vi "Receive Signal DBL.vi"(8 "error in":errorcluster, 10 "Signal Name":string, 11 "DBC Communication in":refnum<class "DBC Communicator.lvclass">) -> (0 "error out":errorcluster, 1 "Time Stamp":timestamp format="%<%x %.3X>T", 2 "Value":dbl, 3 "DBC Communication out":refnum<class "DBC Communicator.lvclass">)   [LabVIEW 2025, in "DBC Communicator.lvclass"]
uses:
  DBC Communicator.lvclass
  <vilib>/xnet/xnet.llb/XNET Frame Type CAN.ctl
  <vilib>/Utility/miscctls.llb/LVMapReplaceAction.ctl
  c9a96274-a027-4ccf-b481-50e0b552ac68.vi
  <vilib>/Utility/error.llb/Trim Whitespace One-Sided.vi
  c9a96274-a027-4ccf-b481-50e0b552ac68.vi/d4db2432-cc9c-482c-8957-dac855435ef6.vi
  c9a96274-a027-4ccf-b481-50e0b552ac68.vi/86fbf154-bd7b-49a2-8ab2-a837b2a95f24.vi
  c9a96274-a027-4ccf-b481-50e0b552ac68.vi/3b95b01e-1ec2-4565-bcd9-7606a5281010.vi
  c9a96274-a027-4ccf-b481-50e0b552ac68.vi/96a08935-737a-44b2-979c-a81d56408f7e.vi
  c9a96274-a027-4ccf-b481-50e0b552ac68.vi/d4db2432-cc9c-482c-8957-dac855435ef6.vi/6eaecd13-6e48-4772-a921-b51ebdf84d88.vi
  c9a96274-a027-4ccf-b481-50e0b552ac68.vi/d4db2432-cc9c-482c-8957-dac855435ef6.vi/d2d5f2b7-06f4-47f6-971c-049c3fdbb653.vi
  c9a96274-a027-4ccf-b481-50e0b552ac68.vi/3b95b01e-1ec2-4565-bcd9-7606a5281010.vi/6eaecd13-6e48-4772-a921-b51ebdf84d88.vi
  c9a96274-a027-4ccf-b481-50e0b552ac68.vi/3b95b01e-1ec2-4565-bcd9-7606a5281010.vi/d2d5f2b7-06f4-47f6-971c-049c3fdbb653.vi
  c9a96274-a027-4ccf-b481-50e0b552ac68.vi/96a08935-737a-44b2-979c-a81d56408f7e.vi/6eaecd13-6e48-4772-a921-b51ebdf84d88.vi
  c9a96274-a027-4ccf-b481-50e0b552ac68.vi/96a08935-737a-44b2-979c-a81d56408f7e.vi/d2d5f2b7-06f4-47f6-971c-049c3fdbb653.vi
  <vilib>/xnet/xnet.llb/XNET Convert (Frame CAN to Signal).vi
  <vilib>/Comparison/Less/Less Functor/Less Functor.lvclass
  Interfaces/IMessage/IMessage.lvclass
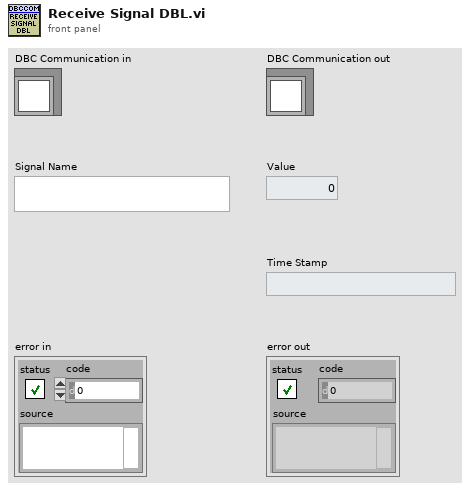
[diagram p1: front panel]
types:
  T1 = typedef "LVMapReplaceAction.ctl" = enum32{"Modify Entry only if found", "Add or Modify Entry", "Delete Entry"}
  T2 = typedef "DBC Communicator.lvclass/ObjectAttributes.ctl" = cluster{"XNET Conversion Session":refnum<k21>, "Frame ID - Timestamp":map{u32, timestamp}, "Signals":cluster{"Names":string[], "Frame IDs":u32[]}}
  T3 = typedef "XNET Frame Type CAN.ctl" = u8
  T4 = cluster{"timestamp":timestamp, "payload":u8[], "identifier":u32, "type":T3, "extended?":bool, "echo?":bool}
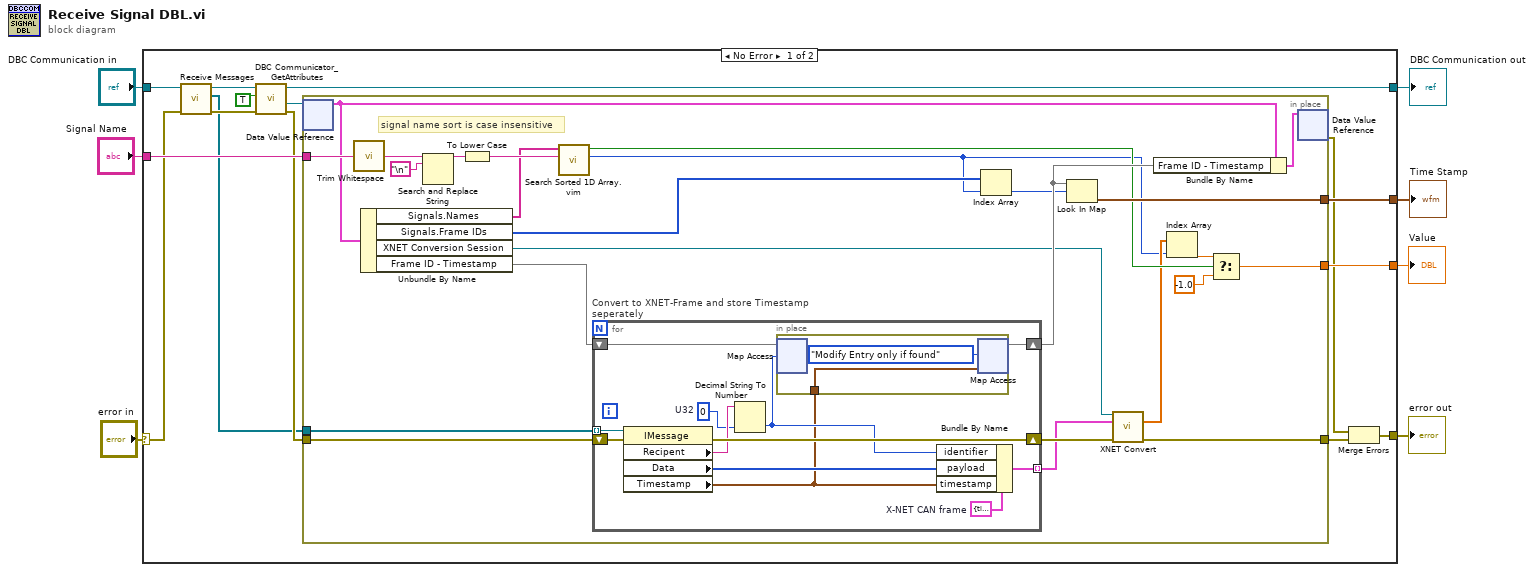
[diagram p0: block diagram]
diagram:
  n1 = case shown="No Error" "error in" {
    selector: "error in" -> [w18 w62]
    tunnel: [w16 w62] -> w6
    tunnel: "Signal Name" -> [w21 _]
    tunnel: [w20 _] -> w4
    tunnel: "DBC Communication in" -> [w11 w63]
    tunnel: [w13 w63] -> w2
    tunnel: [w19 _] -> w1
    frame No Error {
      n2 = call-dynamic "Receive Messages.vi"("Error In"=w18, "Communicator in"=w11) -> ("Error Out"=w12:errorcluster, "Messages"=w9:refnum<class "IMessage.lvclass">[], "Communicator out"=w10:refnum<class "DBC Communicator.lvclass">)  [unwired: 7 in]
      n3 = call "DBC Communicator_GetAttributes.vi"("Error In"=w12, "OnlyGetDvrReference(False)"=TRUE, "reference in"=w10) -> ("Error Out"=w14:errorcluster, "DataRef"=w17:refnum<data-value>, "reference out"=w13:refnum<class "DBC Communicator.lvclass">)  [unwired: 5 in, 1 out]
      n4 = in-place {
        in-place-border: [w47] -> w22
        in-place-border: w21 -> [w46]
        in-place-border: [w45] -> w20
        in-place-border: [w40] -> w19
        in-place-border: w9 -> [w24]
        in-place-border: w14 -> [w23]
        # "signal name sort is case insensitive"
        n5 = in-place-dvr #1(w17) -> (w26:T2)  [unwired: 1 out]
        n6 = call <vilib>:"Trim Whitespace.vi"("string"=w46) -> ("trimmed string"=w29:string)  [unwired: 1 in]
        n7 = Unbundle By Name(w26) -> ("Signals.Names"=w27:string[], "Signals.Frame IDs"=w32:u32[], "XNET Conversion Session"=w39:refnum<k21>, "Frame ID - Timestamp"=w43:map{u32, timestamp})
        n8 = Search and Replace String(input string=w29, search string="\n") -> (result string=w42:string)  [unwired: 6 in, 3 out]
        n9 = To Lower Case(string=w42) -> (all lower case string=w28:string)
        n10 = call "Search Sorted 1D Array.vim"("element"=w28, "sorted 1D array"=w27) -> ("nearest index"=w31:i32, "found?"=w36:bool)  [unwired: 8 in]
        n11 = for "Convert to XNET-Frame and store Timestamp seperately" {
          tunnel: w24 -> [w54] mode=indexing
          shift-right: [w57] -> w38
          shift-left: w23 -> [w53]
          tunnel: [w56] -> w37 mode=indexing
          shift-right: [w48] -> w41
          shift-left: w43 -> [w52]
          w49 = u32 0  # U32
          w59 = T4 {"timestamp"=timestamp(0 s since 1904-01-01), "payload"=[], "identifier"=0, "type"=0, "extended?"=FALSE, "echo?"=FALSE}  # X-NET CAN frame
          n12 = property class="IMessage"(reference=w54, error in=w53) -> (error out=w57:errorcluster, "Recipent"=w55:string, "Data"=w58:u8[], "Timestamp"=w50:timestamp)  [unwired: 1 out]
          n13 = Decimal String To Number(string=w55, default (0L)=w49) -> (number=w51:u32)  [unwired: 1 in, 1 out]
          n14 = in-place {
            in-place-border: w50 -> [w61]
            n15 = in-place-map #2(w52, w51) -> ()  [unwired: 1 in, 2 out]
            n16 = in-place-map #2(w61, LVMapReplaceAction."Modify Entry only if found" ("action")) -> (w48:map{u32, timestamp})  [unwired: 2 out]
          }
          n17 = Bundle By Name(cluster=w59, "identifier"=w51, "payload"=w58, "timestamp"=w50) -> (w56:T4)
        }
        n18 = Index Array(array=w32, index=w31) -> (element=w30:u32)
        n19 = Look In Map(map=w41, key=w30) -> (value=w40:timestamp)  [unwired: 1 in, 1 out]
        n20 = call-poly <vilib>:"XNET Convert.vi"("session in"=w39, "frame data"=w37, "error in (no error)"=w38) -> ("signal data"=w33:dbl[], "error out"=w47:errorcluster)  [unwired: 10 in, 1 out]
        n21 = Bundle By Name(cluster=w26, "Frame ID - Timestamp"=w41) -> (w25:T2)
        n22 = Index Array(array=w33, index=w31) -> (element=w35:dbl)
        n23 = Select(t=w35, s=w36, f=-1.0) -> (s? t:f=w45:dbl)
        n24 = in-place-dvr #1(w25) -> (w15:errorcluster)  [unwired: 1 out]
      }
      n25 = Merge Errors(w15, w22) -> (w16:errorcluster)
    }
    frame Error {
    }
  }
  "error out" <- w6
  "DBC Communication out" <- w2
  "Value" <- w4
  "Time Stamp" <- w1
